vi "Global AllowRead.vi"() -> ()   [LabVIEW 2016]
panel:
  out "Global allow TDC read":bool
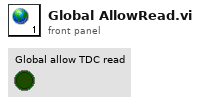
[diagram p1: front panel]
diagram:
